vi "PageUI.vi"() -> ()   [LabVIEW 2019, in "Page.lvclass"]
uses:
  Page.lvclass
  <vilib>/NI/Configuration Framework/Node/NodeRef.ctl
  <vilib>/NI/Configuration Framework/Node/NISE_CEF_Node.lvclass
  <vilib>/NI/AMC/Message Queue.ctl
  <vilib>/NI/AMC/Message.ctl
  <vilib>/NI/Tools/Keyed Array/KeyedArray.ctl
  <vilib>/NI/Configuration Framework/Node/UserEventRef.ctl
  <vilib>/NI/Configuration Framework/Controls/EventCluster.ctl
  System.Windows.Forms
  C:/Program Files (x86)/National Instruments/LabVIEW 2019/vi.lib/NI/Configuration Framework/Node/NISE_CEF_Node.lvclass
  Page.lvclass/Page.ctl
  XML Controls/Help File Properties.ctl
  XML Controls/Path Cluster.ctl
  Read General Page Properties.vi
  Write General Page Properties.vi
  <vilib>/NI/AMC/Create Single Message.vi
  <vilib>/NI/AMC/Update Message Routing Info.vi
  <vilib>/NI/AMC/Send Message.vi
  <vilib>/NI/AMC/AMC.lvlib
  Configuration Tool.lvlib
  VeriStand Custom Device XML Parser.lvlib
  <vilib>/NI/Tools/Keyed Array/Tools_KeyedArray.lvlib
  <vilib>/NI/Configuration Framework/NISE_CEF_TreeControl.lvlib
panel:
  in  "Main UI Tab":T1(tab)
  in  "Glyph":refnum<k24>(container)
  in  "Show Documentation":bool
  in  "Page Name":string
  in  "GUID":string="9b525fa0-4d4a-4ec1-902b-bfeef88ebbcc"
  in  "Host Path to Page VI":path
  in  "Host Path to Glyph":path
  in  "Broken Glyph":refnum<k24>(container)
  in  "Inactive Glyph":refnum<k24>(container)
  in  "Host Path to Inactive Glyph":path
  in  "Host Path to Broken Glyph":path
  in  "Rename":bool
  in  "Delete":bool
  in  "Alphabetical":bool
  in  "Multiselect":bool
  in  "Copy Action":enum16{"copy", "disabled"}(ring)
  in  "Paste Action":T2(ring)
  in  "Host Path to Help File":path
  in  "Help File Type":enum16{"chm", "other"}(ring)
  in  "Help Section":string
  in  "user event":T3
  in  "main queue":T4
  in  "node ref":T5
  # "General Settings"
  # "Page Settings"
  # "Glyph Settings"
  # "Inactive Glyph Settings"
  # "Protection Settings"
  # "Broken Glyph Settings"
  # "Copy/Paste Settings"
  # "Help File Settings"
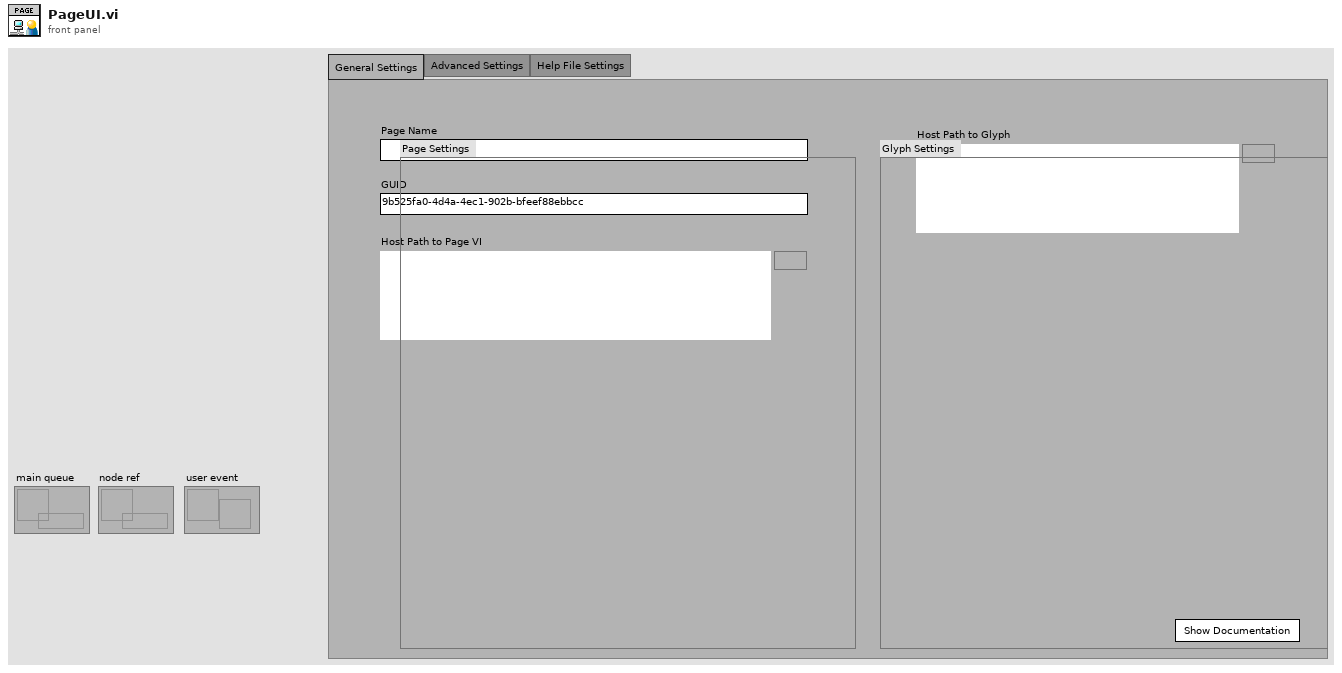
[diagram p1: front panel]
types:
  T1 = enum32{"General Settings", "Advanced Settings", "Help File Settings"}
  T2 = enum16{"Create", "CreatIfNotExists_GUID", "CreatIfNotExists_Name", "Replace", "Dialog"}
  T3 = typedef "NISE_CEF_Node.lvclass/UserEventRef.ctl" = refnum<user-event>
  T4 = typedef "AMC.lvlib/Message Queue.ctl" = refnum<queue>
  T5 = typedef "NISE_CEF_Node.lvclass/NodeRef.ctl" = refnum<data-value>
  T6 = typedef "VeriStand Custom Device XML Parser.lvlib/Page Properties.ctl" = cluster{"Name":string, "Disallow Renaming":bool, "Delete Protection":bool, "Exlcude from Alphabetical order":bool, "Allow Multi-Selection":bool, "GUID":string, "Parent GUIDs":string[], "Glyph":T7, "Inactive Glyph":T7, "Broken Glyph":T7, "Item to Launch":T7, "Additional Information":string, "Copy":enum16{"copy", "disabled"}, "Paste":enum16{"Create", "CreatIfNotExists_GUID", "CreatIfNotExists_Name", "Replace", "Dialog"}, "Help":T8}
  T7 = typedef "VeriStand Custom Device XML Parser.lvlib/Path Cluster.ctl" = cluster{"Path":path, "Path Type":enum16{"Absolute", "To Base", "To Common Doc Dir", "To Application Data Dir"}}
  T8 = typedef "VeriStand Custom Device XML Parser.lvlib/Help File Properties.ctl" = cluster{"Item to Launch":T7, "Section":string, "File Type":enum16{"chm", "other"}}
  T9 = enum16{"Absolute", "To Base", "To Common Doc Dir", "To Application Data Dir"}
  T10 = cluster{path, "VS Enum Out":enum16{"Absolute", "To Base", "To Common Doc Dir", "To Application Data Dir"}}
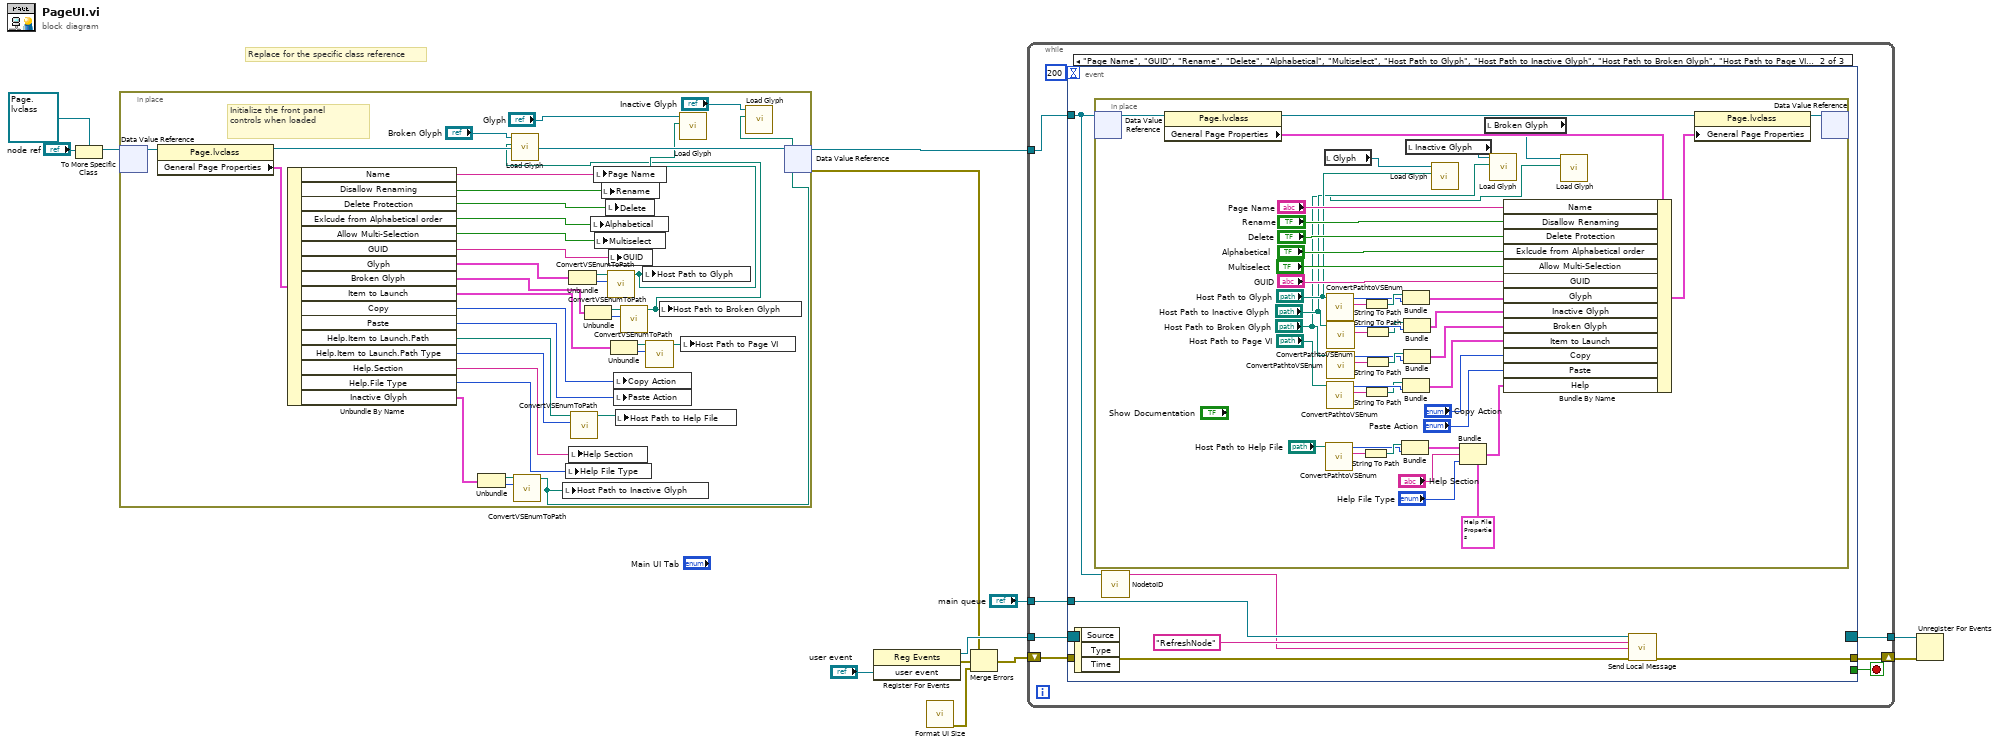
[diagram p0: block diagram]
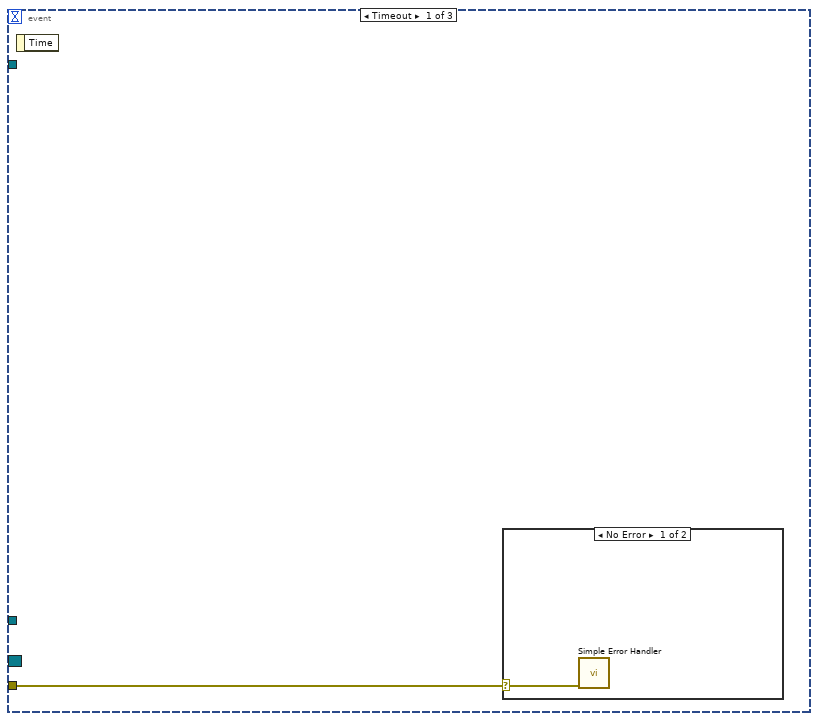
[diagram p2: hidden frame]
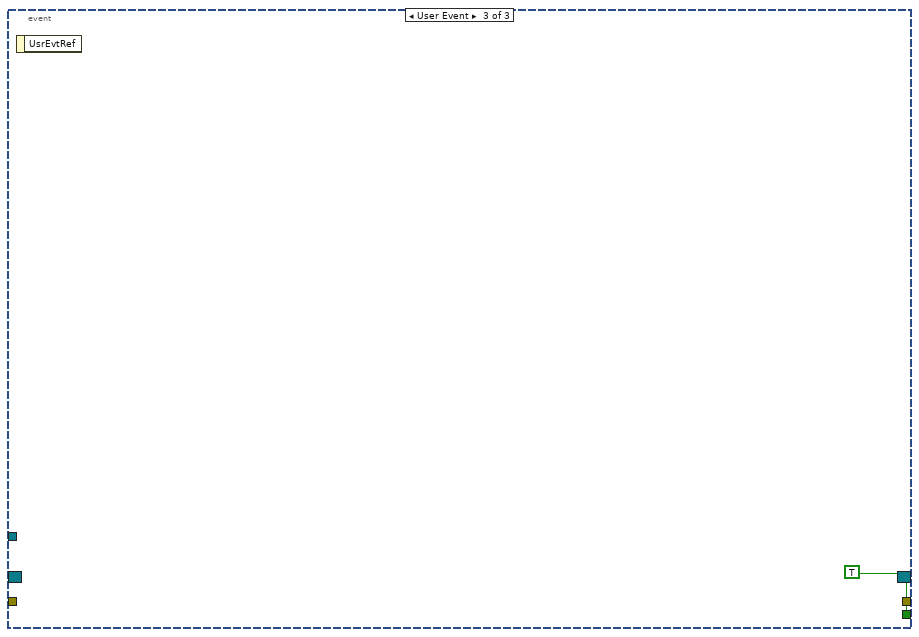
[diagram p4: hidden frame]
diagram:
  # "Replace for the specific class reference"
  n1 = To More Specific Class(target class=refnum<data-value> refnum ("data value reference"), reference="node ref") -> (specific class reference=w6:refnum<data-value>)  [unwired: 1 in, 1 out]
  n2 = in-place {
    # "Initialize the front panel controls when loaded"
    n3 = in-place-dvr #1(w6) -> (w48:refnum<class "Page.lvclass">)  [unwired: 1 out]
    n4 = property class="Page.lvclass"(reference=w48) -> (reference out=w47:refnum<class "Page.lvclass">, "General Page Properties"=w46:T6)  [unwired: 1 in, 1 out]
    n5 = Unbundle By Name(w46) -> ("Name"=w45:string, "Disallow Renaming"=w44:bool, "Delete Protection"=w43:bool, "Exlcude from Alphabetical order"=w42:bool, "Allow Multi-Selection"=w41:bool, "GUID"=w40:string, "Glyph"=w25:T7, "Broken Glyph"=w38:T7, "Item to Launch"=w36:T7, "Copy"=w32:enum16{"copy", "disabled"}, "Paste"=w31:T2, "Help.Item to Launch.Path"=w30:path, "Help.Item to Launch.Path Type"=w29:T9, "Help.Section"=w27:string, "Help.File Type"=w26:enum16{"chm", "other"}, "Inactive Glyph"=w24:T7)
    n6 = Unbundle(w24) -> ("Path"=w23:path, "Path Type"=w22:T9)
    n7 = call "ConvertVSEnumToPath.vi"("Source.Path Type"=w22, "Path In"=w23) -> ("appended path"=w17:path)  [unwired: 9 in]
    n8 = local write "Host Path to Inactive Glyph"(w17) -> ()
    n9 = local write "Help File Type"(w26) -> ()
    n10 = Unbundle(w25) -> ("Path"=w19:path, "Path Type"=w20:T9)
    n11 = local write "Help Section"(w27) -> ()
    n12 = call "ConvertVSEnumToPath.vi"("Source.Path Type"=w29, "Path In"=w30) -> ("appended path"=w28:path)  [unwired: 9 in]
    n13 = Unbundle(w38) -> ("Path"=w33:path, "Path Type"=w39:T9)
    n14 = local write "Alphabetical"(w42) -> ()
    n15 = local write "Page Name"(w45) -> ()
    n16 = local write "Multiselect"(w41) -> ()
    n17 = local write "Rename"(w44) -> ()
    n18 = local write "Delete"(w43) -> ()
    n19 = call "ConvertVSEnumToPath.vi"("Source.Path Type"=w20, "Path In"=w19) -> ("appended path"=w21:path)  [unwired: 9 in]
    n20 = local write "GUID"(w40) -> ()
    n21 = Unbundle(w36) -> ("Path"=w35:path, "Path Type"=w37:T9)
    n22 = local write "Copy Action"(w32) -> ()
    n23 = local write "Paste Action"(w31) -> ()
    n24 = local write "Host Path to Help File"(w28) -> ()
    n25 = call "ConvertVSEnumToPath.vi"("Source.Path Type"=w39, "Path In"=w33) -> ("appended path"=w14:path)  [unwired: 9 in]
    n26 = call "Load Glyph.vi"("Path"=w14, "PictureBox in"="Broken Glyph") -> ()  [unwired: 8 in, 2 out]
    n27 = local write "Host Path to Glyph"(w21) -> ()
    n28 = call "ConvertVSEnumToPath.vi"("Source.Path Type"=w37, "Path In"=w35) -> ("appended path"=w34:path)  [unwired: 9 in]
    n29 = local write "Host Path to Broken Glyph"(w14) -> ()
    n30 = call "Load Glyph.vi"("Path"=w21, "PictureBox in"="Glyph") -> ()  [unwired: 8 in, 2 out]
    n31 = local write "Host Path to Page VI"(w34) -> ()
    n32 = call "Load Glyph.vi"("Path"=w17, "PictureBox in"="Inactive Glyph") -> ()  [unwired: 8 in, 2 out]
    n33 = in-place-dvr #1(w47) -> (w13:refnum<data-value>, w3:errorcluster)
  }
  n34 = register-events("user event") -> (reference out=w10:refnum<event-registration>, error out=w4:errorcluster)  [unwired: 2 in]
  n35 = call "Format UI Size.vi"() -> ("error out"=w1:errorcluster)  [unwired: 11 in]
  n36 = Merge Errors(w3, w4, w1) -> (w2:errorcluster)
  n37 = while {
    tunnel: w13 -> [w56]
    tunnel: "main queue" -> [w55]
    tunnel: w10 -> [w53]
    tunnel: [w52] -> w9
    shift-right: [w50] -> w8
    shift-left: w2 -> [w49]
    stop <- w51 stop-if-true
    n38 = event shown="[1] \"Page Name\", \"GUID\", \"Rename\", \"Delete\", \"Alphabetical\", \"Multiselect\", \"Host Path to Glyph\", \"Host Path to Inactive Glyph\", \"Host Path to Broken Glyph\", \"Host Path to Page VI\", \"Copy Action\", \"Paste Action\", \"Host Path to Help File\", \"Help File Type\", \"Help Section\": Value Change" {
      selector: w53 -> [_ _ _]
      dyn-events: [_ _ _] -> w52
      timeout: 200 -> [_ _ _]
      tunnel: w56 -> [_ w62 _]
      tunnel: w55 -> [_ w63 _]
      tunnel: [_ _ TRUE] -> w51
      tunnel: [_ w60 _] -> w50
      tunnel: w49 -> [w57 w59 _]
      event Timeout {
        n39 = event-data() -> ()  [unwired: 1 in, 1 out]
        n40 = case shown="No Error" w57 {
          selector: w57 -> [w58 _]
          frame No Error {
            n41 = call <vilib>:"Simple Error Handler.vi"("error in (no error)"=w58) -> ()  [unwired: 4 in, 5 out]
          }
          frame Error {
          }
        }
      }
      event "Page Name", "GUID", "Rename", "Delete", "Alphabetical", "Multiselect", "Host Path to Glyph", "Host Path to Inactive Glyph", "Host Path to Broken Glyph", "Host Path to Page VI", "Copy Action", "Paste Action", "Host Path to Help File", "Help File Type", "Help Section": Value Change {
        n42 = event-data() -> ()  [unwired: 1 in, 3 out]
        n43 = in-place {
          n44 = in-place-dvr #2(w62) -> (w108:refnum<class "Page.lvclass">)  [unwired: 1 out]
          n45 = property class="Page.lvclass"(reference=w108) -> (reference out=w107:refnum<class "Page.lvclass">, "General Page Properties"=w106:T6)  [unwired: 1 in, 1 out]
          n46 = local read "Glyph"() -> (w70:refnum<k24>)
          n47 = call "ConvertPathtoVSEnum.vi"("Path In"="Host Path to Help File") -> ("Remaining Path"=w80:string, "VS Enum Out"=w78:T9)  [unwired: 9 in]
          n48 = call "ConvertPathtoVSEnum.vi"("Path In"="Host Path to Glyph") -> ("Remaining Path"=w98:string, "VS Enum Out"=w96:T9)  [unwired: 9 in]
          n49 = call "ConvertPathtoVSEnum.vi"("Path In"="Host Path to Page VI") -> ("Remaining Path"=w87:string, "VS Enum Out"=w89:T9)  [unwired: 9 in]
          n50 = call "ConvertPathtoVSEnum.vi"("Path In"="Host Path to Inactive Glyph") -> ("Remaining Path"=w93:string, "VS Enum Out"=w95:T9)  [unwired: 9 in]
          n51 = call "ConvertPathtoVSEnum.vi"("Path In"="Host Path to Broken Glyph") -> ("Remaining Path"=w92:string, "VS Enum Out"=w90:T9)  [unwired: 9 in]
          n52 = String To Path(string=w80) -> (path=w79:path)
          n53 = String To Path(string=w98) -> (path=w97:path)
          n54 = String To Path(string=w87) -> (path=w88:path)
          n55 = String To Path(string=w93) -> (path=w94:path)
          n56 = String To Path(string=w92) -> (path=w91:path)
          n57 = Bundle(w79, "VS Enum Out"=w78) -> (w76:T10)  [unwired: 1 in]
          n58 = Bundle(w97, "VS Enum Out"=w96) -> (w99:T10)  [unwired: 1 in]
          n59 = Bundle(w88, "VS Enum Out"=w89) -> (w83:T10)  [unwired: 1 in]
          n60 = Bundle(w94, "VS Enum Out"=w95) -> (w86:T10)  [unwired: 1 in]
          n61 = Bundle(w91, "VS Enum Out"=w90) -> (w85:T10)  [unwired: 1 in]
          n62 = local read "Inactive Glyph"() -> (w69:refnum<k24>)
          n63 = call "Load Glyph.vi"("Path"="Host Path to Glyph", "PictureBox in"=w70) -> ()  [unwired: 8 in, 2 out]
          n64 = Bundle(cluster=T8 {"Item to Launch"={"Path"=path "", "Path Type"=enum."Absolute"}, "Section"="", "File Type"=enum."chm"} ("Help"), "Item to Launch"=w76, "Section"="Help Section", "File Type"="Help File Type") -> (w72:T8)
          n65 = local read "Broken Glyph"() -> (w68:refnum<k24>)
          n66 = call "Load Glyph.vi"("Path"="Host Path to Inactive Glyph", "PictureBox in"=w69) -> ()  [unwired: 8 in, 2 out]
          n67 = Bundle By Name(cluster=w106, "Name"="Page Name", "Disallow Renaming"="Rename", "Delete Protection"="Delete", "Exlcude from Alphabetical order"="Alphabetical", "Allow Multi-Selection"="Multiselect", "GUID"="GUID", "Glyph"=w99, "Inactive Glyph"=w86, "Broken Glyph"=w85, "Item to Launch"=w83, "Copy"="Copy Action", "Paste"="Paste Action", "Help"=w72) -> (w71:T6)
          n68 = call "Load Glyph.vi"("Path"="Host Path to Broken Glyph", "PictureBox in"=w68) -> ()  [unwired: 8 in, 2 out]
          n69 = property class="Page.lvclass"(reference=w107, "General Page Properties"=w71) -> (reference out=w109:refnum<class "Page.lvclass">)  [unwired: 1 in, 1 out]
          n70 = in-place-dvr #2(w109) -> ()  [unwired: 2 out]
        }
        n71 = call <vilib>:"NodetoID.vi"("node ref"=w62) -> ("ID"=w61:string)  [unwired: 9 in, 1 out]
        n72 = call <vilib>:"Send Local Message.vi"("message queue in"=w63, "message name"="RefreshNode" ("Message Name"), "message value"=w61, "error in"=w59) -> ("error out"=w60:errorcluster)  [unwired: 9 in, 2 out]
      }
      event User Event {
        n73 = event-data() -> ()  [unwired: 1 in, 1 out]
      }
    }
  }
  n74 = Unregister For Events(event registration refnum=w9, error in=w8) -> ()  [unwired: 1 out]
